vi "Start Pulse Measurements.vi"(8 "error in (no error)":errorcluster, 9 "Repeat times":i32=1, 10 "Objects":string[](array[string]), 11 "Monitor-Pulse in":refnum<class "Monitor-Pulse.lvclass">) -> (0 "error out":errorcluster, 3 "Monitor-Pulse out":refnum<class "Monitor-Pulse.lvclass">)   [LabVIEW 2015, in "Monitor-Pulse.lvclass"]
uses:
  Monitor-Pulse.lvclass
  Measure_core/Measure Controller Messages/Result Response Msg/Result Response Msg.lvclass
  <vilib>/ActorFramework/Actor/Actor.lvclass/Actor.ctl
  <vilib>/ActorFramework/Message Enqueuer/Message Enqueuer.lvclass/Message Enqueuer.ctl
  Measure_core/Measure Object Messages/Self-Addressed Msg/Self-addressed Msg.lvclass/Self-addressed Msg.ctl
  Measure_core/Measure Controller Messages/Start Measurements Msg/Start Measurements Msg.lvclass/Start Measurements Msg.ctl
  Measure_core/Measure Object Messages/Self-Addressed Msg/Write Return Enqueuer.vi
  <vilib>/ActorFramework/Message Enqueuer/Init from Existing Queue.vi
  <vilib>/ActorFramework/Message Enqueuer/Enqueue.vi
  <vilib>/ActorFramework/Message Priority Queue/Priority Enqueue.vi
  <vilib>/ActorFramework/Message Enqueuer/Message Enqueuer.lvclass
  Measure_core/Measure Controller Messages/Start Measurements Msg/Start Measurements Msg.lvclass
  <vilib>/ActorFramework/Actor/Actor.lvclass
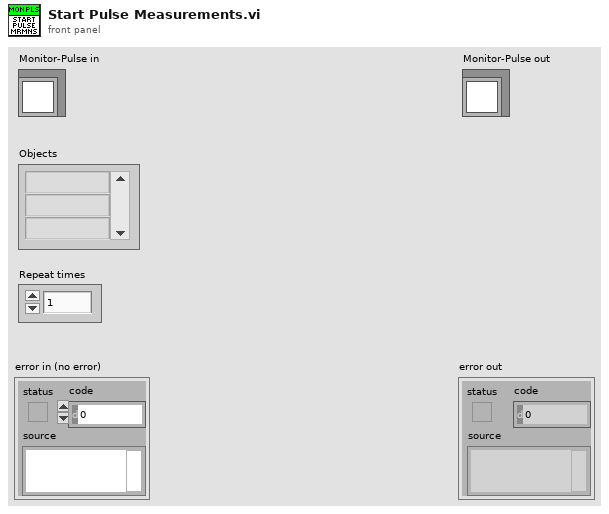
[diagram p1: front panel]
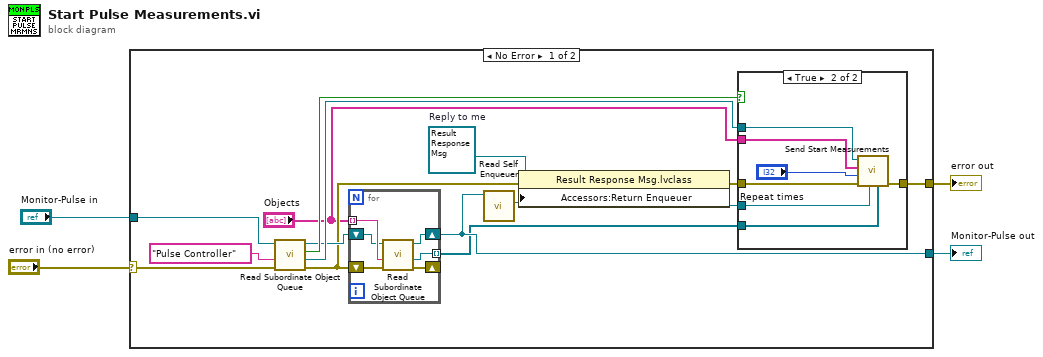
[diagram p0: block diagram]
diagram:
  n1 = case shown="No Error" "error in (no error)" {
    selector: "error in (no error)" -> [w14 w35]
    tunnel: [w16 w35] -> w3
    tunnel: [w9 w34] -> w1
    tunnel: "Monitor-Pulse in" -> [w15 w34]
    frame No Error {
      w5 = refnum<class "Result Response Msg.lvclass"> refnum  # Reply to me
      n2 = call-dynamic "Read Subordinate Object Queue.vi"("error in (no error)"=w14, "Name"="Pulse Controller", "Measure Object in"=w15) -> ("error out"=w8:errorcluster, "Object Enqueuer"=w18:refnum<class "Message Enqueuer.lvclass">, "Found?"=w17:bool, "Measure Object out"=w10:refnum<class "Monitor-Pulse.lvclass">)  [unwired: 5 in]
      n3 = for {
        tunnel: "Objects" -> [w25] mode=indexing
        shift-right: [w23] -> w9
        shift-left: w10 -> [w24]
        shift-right: [w21] -> _
        shift-left: w8 -> [w22]
        tunnel: [w20] -> w7 mode=indexing
        n4 = call-dynamic "Read Subordinate Object Queue.vi"("error in (no error)"=w22, "Name"=w25, "Measure Object in"=w24) -> ("error out"=w21:errorcluster, "Object Enqueuer"=w20:refnum<class "Message Enqueuer.lvclass">, "Measure Object out"=w23:refnum<class "Monitor-Pulse.lvclass">)  [unwired: 5 in, 1 out]
      }
      n5 = call <vilib>:"Read Self Enqueuer.vi"("Actor"=w9) -> ("Self Enqueuer"=w13:refnum<class "Message Enqueuer.lvclass">)  [unwired: 10 in]
      n6 = property class="Result Response Msg.lvclass"(reference=w5, error in=w8, "Accessors:Return Enqueuer"=w13) -> (reference out=w12:refnum<class "Result Response Msg.lvclass">, error out=w11:errorcluster)
      n7 = case shown="True" w17 {
        tunnel: w18 -> [_ w33]
        tunnel: w11 -> [w26 w32]
        tunnel: [w26 w30] -> w16
        tunnel: w12 -> [_ w29]
        tunnel: w7 -> [_ w28]
        tunnel: "Objects" -> [_ w27]
        frame False {
        }
        frame True {
          n8 = call "Send Start Measurements.vi"("Objects enqueuers"=w28, "Reply to"=w29, "error in (no error)"=w32, "Repeat times"="Repeat times", "Objects"=w27, "Message Enqueuer"=w33) -> ("error out"=w30:errorcluster)  [unwired: 4 in, 1 out]
        }
      }
    }
    frame Error {
    }
  }
  "error out" <- w3
  "Monitor-Pulse out" <- w1
